vi "64Out_2 OutBit.vi"(8 "error in (no error)":errorcluster, 10 "BL":bool, 11 "IO_Output_2 Select":T1=enum."汽缸降_6#移載三") -> (0 "error out":errorcluster)   [LabVIEW 2019]
uses:
  Ctrl/64Out_2 SelectOut.ctl
  global/IO_ClassTypeData.vi
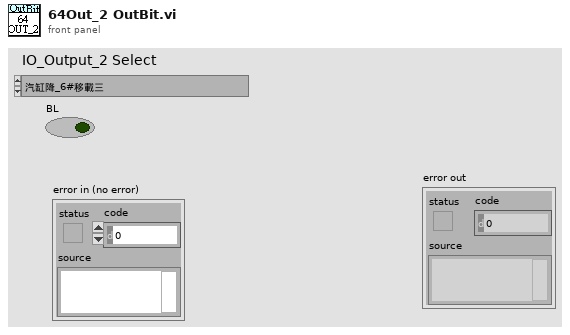
[diagram p1: front panel]
types:
  T1 = typedef "64Out_2 SelectOut.ctl" = enum16{"移入軌道氣缸#模組七", "軌道分料氣缸#模組七", "移入旋轉台氣缸#模組七", "旋轉台氣缸#模組七", "收料燈號#模組七", "UBE#2", "汽缸升_1#移載一", "汽缸降_1#移載一", "汽缸升_2#移載一", "汽缸降_2#移載一", "放料汽缸_1#移載一", "放料汽缸_2#移載一", "汽缸升_3#移載二", "汽缸降_3#移載二", "汽缸升_4#移載二", "汽缸降_4#移載二", "放料汽缸_3#移載二", "放料汽缸_4#移載二", "汽缸升_5#移載三", "汽缸降_5#移載三", "汽缸升_6#移載三", "汽缸降_6#移載三", "放料汽缸_5#移載三", "放料汽缸_6#移載三", "汽缸升_7#移載四", "汽缸降_7#移載四", "放料汽缸_7#移載四", "UBE#10", "綠", "黃", "紅", "嗡鳴器", "UBE#15", "UBE#16", "UBE#17", "UBE#18", "UBE#19", "UBE#20", "UBE#21", "UBE#22", "UBE#23", "UBE#24", "UBE#25", "UBE#26", "UBE#27", "UBE#28", "UBE#29", "UBE#30", "UBE#31", "UBE#32", "UBE#33", "UBE#34", "UBE#35", "UBE#36", "UBE#37", "UBE#38", "UBE#39", "UBE#40", "UBE#41", "UBE#42", "UBE#43", "UBE#44", "UBE#45", "UBE#46"}
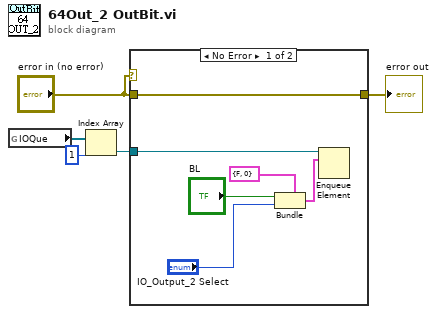
[diagram p0: block diagram]
diagram:
  n1 = global read "IO_ClassTypeData.vi" "IOQue"() -> (w3:refnum<queue>[])
  n2 = Index Array(array=w3, index=1) -> (element=w2:refnum<queue>)
  n3 = case shown="No Error" "error in (no error)" {
    tunnel: "error in (no error)" -> [w6 w12]
    tunnel: [w6 w12] -> w5
    tunnel: w2 -> [w11 _]
    frame No Error {
      n4 = Bundle(cluster=cluster{"BL":bool, "Index":i32} {"BL"=FALSE, "Index"=0} ("element"), "BL"="BL", "Index"="IO_Output_2 Select") -> (w8:cluster{"BL":bool, "Index":i32})
      n5 = Enqueue Element(queue=w11, element=w8) -> ()  [unwired: 2 in, 3 out]
    }
    frame Error {
    }
  }
  "error out" <- w5
